vi "Generate PWM.vi"(6 "sampling info":cluster{"Fs":dbl, "#s":dbl}={"Fs"=1000.0, "#s"=1000.0} {"Fs" format="%.2p"}, 7 "reset?":bool, 8 "error in":errorcluster, 10 "duty cycle":dbl=50.0 format="%0.2f", 11 "frequency":dbl=10.0 format="%0.2p") -> (0 "error out":errorcluster, 2 "digital waveform":digitalwaveform(waveform)={"t0"=timestamp(0 s since 1904-01-01), "dt"=0.0, "Y"={"transitions"=[], "data"=[]}, "error"={"status"=FALSE, "code"=37421928, "source"=""}})   [LabVIEW 2024]
uses:
  <vilib>/Waveform/DWDTOps.llb/DWDT Boolean Array to Digital.vi
  <vilib>/measure/NI_MABase.lvlib
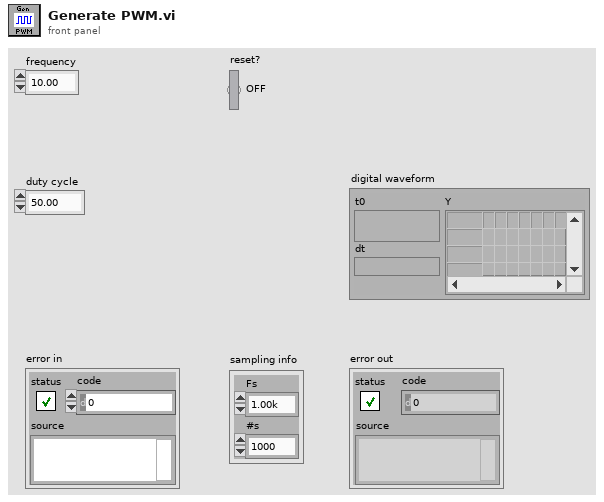
[diagram p1: front panel]
types:
  T1 = enum16{"Sine Wave", "Triangle Wave", "Square Wave", "Sawtooth Wave"}
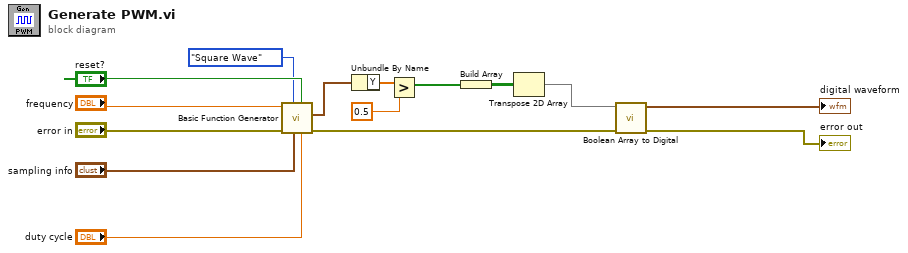
[diagram p0: block diagram]
diagram:
  n1 = call <vilib>:"Basic Function Generator.vi"("square wave duty cycle (%)"="duty cycle", "reset signal"="reset?", "sampling info"="sampling info", "signal type"=T1."Square Wave", "error in (no error)"="error in", "frequency"="frequency") -> ("error out"=w4:errorcluster, "signal out"=w3:waveform(dbl))  [unwired: 3 in, 1 out]
  n2 = Unbundle By Name(w3) -> ("Y"=w7:dbl[])
  n3 = Greater?(x=w7, y=0.5) -> (0:w5:bool[])
  n4 = Build Array(w5) -> (w2:bool[][])
  n5 = Transpose 2D Array(2D array=w2) -> (transposed array=w1:bool[][])
  n6 = call-poly <vilib>:"Boolean Array to Digital.vi"("error in (no error)"=w4, "boolean array"=w1) -> ("error out"=→"error out":errorcluster, "digital waveform"=→"digital waveform":digitalwaveform)  [unwired: 8 in]
